vi "Check id.vi"(9 "password":string, 10 "user name":string, 11 "users in":T1(array[cluster])) -> (1 "id ok":bool, 2 "first access":bool, 3 "users out":T1(array[cluster]), 5 "permission":string)   [LabVIEW 2018]
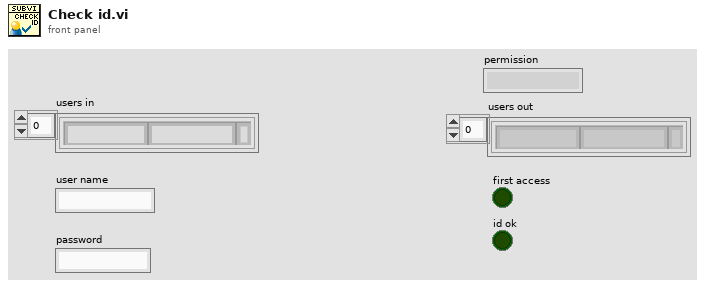
[diagram p1: front panel]
types:
  T1 = cluster{"name":string, "permission":string, "password":string}[]
  T2 = cluster{"name":string, "permission":string, "password":string}
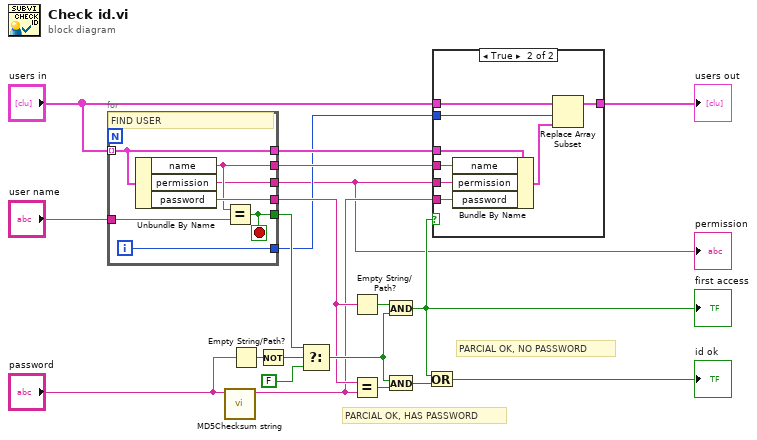
[diagram p0: block diagram]
diagram:
  # "PARCIAL OK, NO PASSWORD"
  # "PARCIAL OK, HAS PASSWORD"
  n1 = for {
    tunnel: "users in" -> [w22] mode=indexing
    tunnel: "user name" -> [w27]
    tunnel: [w26] -> w18
    tunnel: [w25] -> w12
    tunnel: [w24] -> w11
    tunnel: [w23] -> w5
    tunnel: [w22] -> w10
    tunnel: [w21] -> w8
    i -> [w21]
    stop <- w26 stop-if-true
    # "FIND USER"
    n2 = Unbundle By Name(w22) -> ("name"=w24:string, "permission"=w23:string, "password"=w25:string)
    n3 = Equal?(x=w24, y=w27) -> (x = y?=w26:bool)
  }
  "permission" <- w5
  n4 = call <vilib>:"MD5Checksum string.vi"("Message String"="password") -> ("MD5 message-digest"=w9:string)  [unwired: 10 in]
  n5 = Empty String/Path?(string/path="password") -> (empty?=w19:bool)
  n6 = Not(x=w19) -> (.not. x?=w20:bool)
  n7 = Select(t=w18, s=w20, f=FALSE) -> (s? t:f=w13:bool)
  n8 = Empty String/Path?(string/path=w12) -> (empty?=w15:bool)
  n9 = Equal?(x=w12, y=w9) -> (x = y?=w14:bool)
  n10 = And(x=w15, y=w13) -> (x .and. y?=w6:bool)
  "first access" <- w6
  n11 = And(x=w13, y=w14) -> (x .and. y?=w16:bool)
  n12 = Or(x=w6, y=w16) -> (x .or. y?=→"id ok":bool)
  n13 = case shown="True" w6 {
    tunnel: w11 -> [_ w35]
    tunnel: w5 -> [_ w34]
    tunnel: "users in" -> [w28 w32]
    tunnel: w10 -> [_ w36]
    tunnel: w9 -> [_ w33]
    tunnel: w8 -> [_ w30]
    tunnel: [w28 w29] -> w3
    frame False {
    }
    frame True {
      n14 = Bundle By Name(cluster=w36, "name"=w35, "permission"=w34, "password"=w33) -> (w31:T2)
      n15 = Replace Array Subset(array=w32, new element=w31, index=w30) -> (w29:T1)
    }
  }
  "users out" <- w3
